vi "FindVISAResource.vi"(8 "error in (no error)":errorcluster) -> (0 "error out":errorcluster, 3 "串口配置Out":T1={"端口选择"=" ", "波特率"=115200, "数据位"=8, "奇偶校验"=0, "停止位"=10, "流控"=0} {"流控" items=["None"=0, "XON/XOFF"=1, "RTS/CTS"=2, "DTR/DSR"=4]; "停止位" items=["1.0"=10, "1.5"=15, "2.0"=20]; "奇偶校验" items=["None", "Odd", "Even", "Mark", "Space"]; "数据位" min=5 max=8 step=1})   [LabVIEW 2015]
uses:
  <vilib>/Utility/miscctls.llb/LVPointTypeDef.ctl
  <vilib>/Instr/_visa.llb/VISA Find Search Mode.ctl
panel:
  in  "串口配置Out":T1={"端口选择"="COM2", "波特率"=57600, "数据位"=8, "奇偶校验"=0, "停止位"=10, "流控"=0} {"流控" items=["None"=0, "XON/XOFF"=1, "RTS/CTS"=2, "DTR/DSR"=4]; "停止位" items=["1.0"=10, "1.5"=15, "2.0"=20]; "奇偶校验" items=["None", "Odd", "Even", "Mark", "Space"]; "数据位" min=5 max=8 step=1}
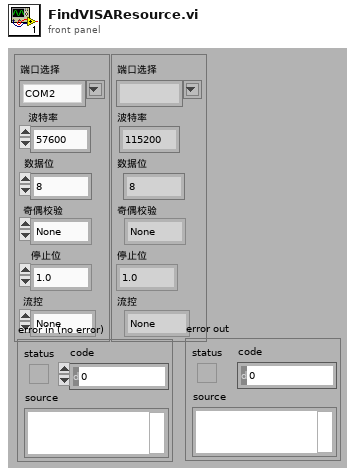
[diagram p1: front panel]
types:
  T1 = cluster{"端口选择":string, "波特率":u32, "数据位":u16, "奇偶校验":u16, "停止位":u16, "流控":u16}
  T2 = typedef "LVPointTypeDef.ctl" = cluster{"Horizontal":i16, "Vertical":i16}
  T3 = typedef "VISA Find Search Mode.ctl" = u32
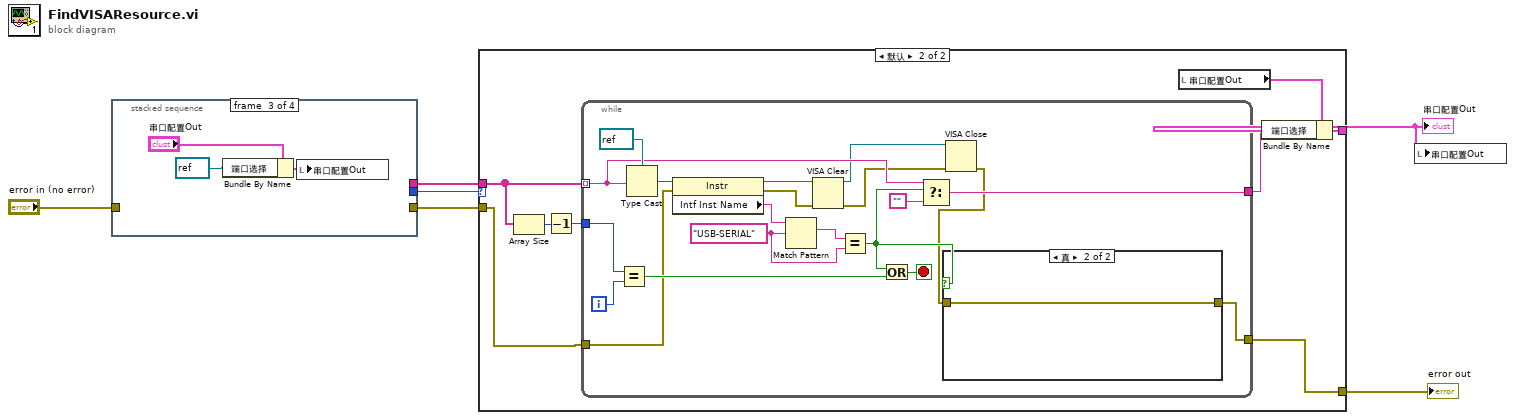
[diagram p0: block diagram]
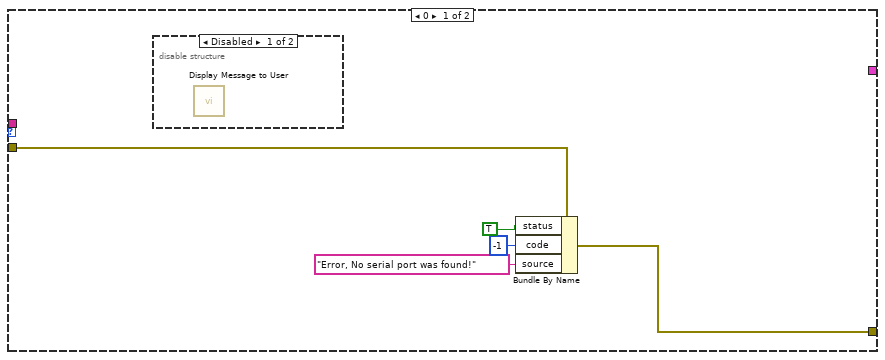
[diagram p2: hidden frame]
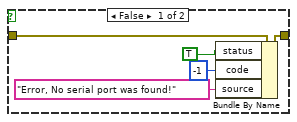
[diagram p4: hidden frame]
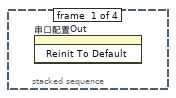
[diagram p5: hidden frame]
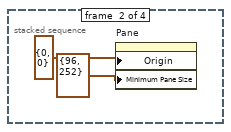
[diagram p6: hidden frame]
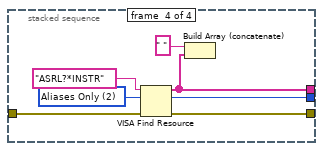
[diagram p7: hidden frame]
diagram:
  n1 = stacked-sequence {
    tunnel: [_ _ _ w15] -> w5
    tunnel: [_ _ _ w14] -> w6
    tunnel: "error in (no error)" -> [_ _ _ w13]
    tunnel: [_ _ _ w12] -> w2
    frame #0 {
      n2 = invoke on="串口配置Out" class="Clust (strict)" method="Reinit To Default"() -> ()  [unwired: 3 in, 3 out]
    }
    frame #1 {
      n3 = property on="Pane" class="Pane"("Origin"=T2 {"Horizontal"=0, "Vertical"=0}, "Minimum Pane Size"=T2 {"Horizontal"=96, "Vertical"=252}) -> ()  [unwired: 2 in, 2 out]
    }
    frame #2 {
      n4 = Bundle By Name(cluster="串口配置Out", "端口选择"=refnum<visa-resource-name> refnum ("COM")) -> (w10:T1)
      n5 = local write "串口配置Out"(w10) -> ()
    }
    frame #3 {
      w18 = T3 2 items=["Canonical Names Only"=0, "Aliases Only"=2, "Include Matching Aliases"=3, "Include All Aliases"=4] ("Search Mode")
      n6 = VISA Find Resource(8:w13, 10:w18, 11:"ASRL?*INSTR" ("expression (\"?*\")")) -> (0:w12:errorcluster, 2:w15:u32, 3:w14:string[])
      n7 = Build Array (concatenate)(" " ("expression (\"?*\")"), w14) -> ()  [unwired: 1 out]
    }
  }
  n8 = case shown="默认" w5 {
    tunnel: w6 -> [_ w31]
    tunnel: [_ w26] -> w4
    tunnel: w2 -> [w23 w25]
    tunnel: [w21 w24] -> w1
    frame 0 {
      n9 = disable-structure shown="Disabled" {
        frame Disabled {
          n10 = call "Display Message to User"() -> ()  [unwired: 3 in, 9 out]
        }
        frame Enabled {
        }
      }
      n11 = Bundle By Name(cluster=w23, "status"=TRUE, "code"=-1, "source"="Error, No serial port was found!") -> (w21:errorcluster)
    }
    frame Default {
      n12 = Array Size(array=w31) -> (size(s)=w30:i32)
      n13 = Decrement(x=w30) -> (x-1=w29:i32)
      n14 = while {
        tunnel: w31 -> [w43] mode=indexing
        tunnel: w29 -> [w45]
        tunnel: [w41] -> w27
        tunnel: w25 -> [w33]
        tunnel: [w34] -> w24
        i -> [w46]
        stop <- w44 stop-if-true
        w47 = "USB-SERIAL" ("regular expression")
        n15 = Equal?(x=w45, y=w46) -> (x = y?=w36:bool)
        n16 = Type Cast(type=refnum<visa-resource-name> refnum ("reference"), x=w43) -> (*(type *) &x=w50:refnum<visa-resource-name>)
        n17 = property class="Instr"(reference=w50, error in=w33) -> (reference out=w39:refnum<visa-resource-name>, error out=w38:errorcluster, "Intf Inst Name"=w49:string)
        n18 = Match Pattern(string=w49, regular expression=w47) -> (match substring=w48:string)  [unwired: 4 out]
        n19 = VISA Clear(VISA resource name=w39, error in (no error)=w38) -> (VISA resource name out=w40:refnum<visa-resource-name>, error out=w37:errorcluster)
        n20 = Equal?(x=w48, y=w47) -> (x = y?=w35:bool)
        n21 = Or(x=w35, y=w36) -> (x .or. y?=w44:bool)
        n22 = Select(t=w43, s=w35, f="") -> (s? t:f=w41:string)
        n23 = VISA Close(VISA resource name=w40, error in (no error)=w37) -> (error out=w32:errorcluster)
        n24 = case shown="真" w35 {
          tunnel: w32 -> [w53 w57]
          tunnel: [w52 w57] -> w34
          frame False {
            n25 = Bundle By Name(cluster=w53, "status"=TRUE, "code"=-1, "source"="Error, No serial port was found!") -> (w52:errorcluster)
          }
          frame True {
          }
        }
      }
      n26 = local read "串口配置Out"() -> (w28:T1)
      n27 = Bundle By Name(cluster=w28, "端口选择"=w27) -> (w26:T1)
    }
  }
  "串口配置Out" <- w4
  "error out" <- w1
  n28 = local write "串口配置Out"(w4) -> ()
